vi "FTS Setup Virtual Source.vi"(8 "error in (no error)":errorcluster, 9 "parameters":T1, 10 "type":u16, 11 "specIndex":u16) -> (0 "error out":errorcluster, 1 "parameters out":T1, 3 "function return":i32)   [LabVIEW 2010, in "FTSLib.lvlib"]
doc: "int __cdecl FTS_SetupVirtualSource(unsigned short specIndex, VIRTUAL_SOURCE_TYPE type, virtual_source_parameter_t *parameters);"
uses:
  FTSLib.lvlib
  FTSLib.dll
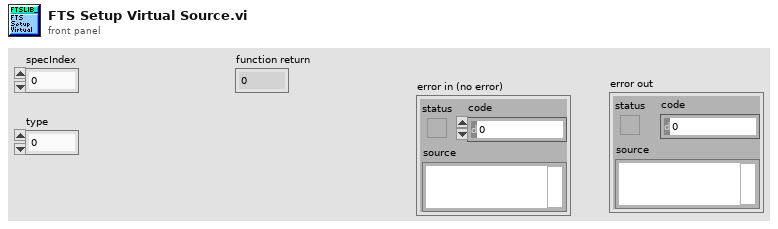
[diagram p1: front panel]
types:
  T1 = cluster{"peakNum":u32, "@dummy control@":i8, "@dummy control@":i8, "@dummy control@":i8, "@dummy control@":i8, "centerWavelength_nm[0]":dbl, "centerWavelength_nm[1]":dbl, "centerWavelength_nm[2]":dbl, "centerWavelength_nm[3]":dbl, "centerWavelength_nm[4]":dbl, "centerWavelength_nm[5]":dbl, "centerWavelength_nm[6]":dbl, "centerWavelength_nm[7]":dbl, "centerWavelength_nm[8]":dbl, "centerWavelength_nm[9]":dbl, "centerWavelength_nm[10]":dbl, "centerWavelength_nm[11]":dbl, "centerWavelength_nm[12]":dbl, "centerWavelength_nm[13]":dbl, "centerWavelength_nm[14]":dbl, "centerWavelength_nm[15]":dbl, "centerWavelength_nm[16]":dbl, "centerWavelength_nm[17]":dbl, "centerWavelength_nm[18]":dbl, "centerWavelength_nm[19]":dbl, "centerWavelength_nm[20]":dbl, "centerWavelength_nm[21]":dbl, "centerWavelength_nm[22]":dbl, "centerWavelength_nm[23]":dbl, "centerWavelength_nm[24]":dbl, "centerWavelength_nm[25]":dbl, "centerWavelength_nm[26]":dbl, "centerWavelength_nm[27]":dbl, "centerWavelength_nm[28]":dbl, "centerWavelength_nm[29]":dbl, "centerWavelength_nm[30]":dbl, "centerWavelength_nm[31]":dbl, "centerWavelength_nm[32]":dbl, "centerWavelength_nm[33]":dbl, "centerWavelength_nm[34]":dbl, "centerWavelength_nm[35]":dbl, "centerWavelength_nm[36]":dbl, "centerWavelength_nm[37]":dbl, "centerWavelength_nm[38]":dbl, "centerWavelength_nm[39]":dbl, "centerWavelength_nm[40]":dbl, "centerWavelength_nm[41]":dbl, "centerWavelength_nm[42]":dbl, "centerWavelength_nm[43]":dbl, "centerWavelength_nm[44]":dbl, "centerWavelength_nm[45]":dbl, "centerWavelength_nm[46]":dbl, "centerWavelength_nm[47]":dbl, "centerWavelength_nm[48]":dbl, "centerWavelength_nm[49]":dbl, "centerWavelength_nm[50]":dbl, "centerWavelength_nm[51]":dbl, "centerWavelength_nm[52]":dbl, "centerWavelength_nm[53]":dbl, "centerWavelength_nm[54]":dbl, "centerWavelength_nm[55]":dbl, "centerWavelength_nm[56]":dbl, "centerWavelength_nm[57]":dbl, "centerWavelength_nm[58]":dbl, "centerWavelength_nm[59]":dbl, "centerWavelength_nm[60]":dbl, "centerWavelength_nm[61]":dbl, "centerWavelength_nm[62]":dbl, "centerWavelength_nm[63]":dbl, "fwhm_nm[0]":dbl, "fwhm_nm[1]":dbl, "fwhm_nm[2]":dbl, "fwhm_nm[3]":dbl, "fwhm_nm[4]":dbl, "fwhm_nm[5]":dbl, "fwhm_nm[6]":dbl, "fwhm_nm[7]":dbl, "fwhm_nm[8]":dbl, "fwhm_nm[9]":dbl, "fwhm_nm[10]":dbl, "fwhm_nm[11]":dbl, "fwhm_nm[12]":dbl, "fwhm_nm[13]":dbl, "fwhm_nm[14]":dbl, "fwhm_nm[15]":dbl, "fwhm_nm[16]":dbl, "fwhm_nm[17]":dbl, "fwhm_nm[18]":dbl, "fwhm_nm[19]":dbl, "fwhm_nm[20]":dbl, "fwhm_nm[21]":dbl, "fwhm_nm[22]":dbl, "fwhm_nm[23]":dbl, "fwhm_nm[24]":dbl, "fwhm_nm[25]":dbl, "fwhm_nm[26]":dbl, "fwhm_nm[27]":dbl, "fwhm_nm[28]":dbl, "fwhm_nm[29]":dbl, "fwhm_nm[30]":dbl, "fwhm_nm[31]":dbl, "fwhm_nm[32]":dbl, "fwhm_nm[33]":dbl, "fwhm_nm[34]":dbl, "fwhm_nm[35]":dbl, "fwhm_nm[36]":dbl, "fwhm_nm[37]":dbl, "fwhm_nm[38]":dbl, "fwhm_nm[39]":dbl, "fwhm_nm[40]":dbl, "fwhm_nm[41]":dbl, "fwhm_nm[42]":dbl, "fwhm_nm[43]":dbl, "fwhm_nm[44]":dbl, "fwhm_nm[45]":dbl, "fwhm_nm[46]":dbl, "fwhm_nm[47]":dbl, "fwhm_nm[48]":dbl, "fwhm_nm[49]":dbl, "fwhm_nm[50]":dbl, "fwhm_nm[51]":dbl, "fwhm_nm[52]":dbl, "fwhm_nm[53]":dbl, "fwhm_nm[54]":dbl, "fwhm_nm[55]":dbl, "fwhm_nm[56]":dbl, "fwhm_nm[57]":dbl, "fwhm_nm[58]":dbl, "fwhm_nm[59]":dbl, "fwhm_nm[60]":dbl, "fwhm_nm[61]":dbl, "fwhm_nm[62]":dbl, "fwhm_nm[63]":dbl, "peakAmplitude[0]":dbl, "peakAmplitude[1]":dbl, "peakAmplitude[2]":dbl, "peakAmplitude[3]":dbl, "peakAmplitude[4]":dbl, "peakAmplitude[5]":dbl, "peakAmplitude[6]":dbl, "peakAmplitude[7]":dbl, "peakAmplitude[8]":dbl, "peakAmplitude[9]":dbl, "peakAmplitude[10]":dbl, "peakAmplitude[11]":dbl, "peakAmplitude[12]":dbl, "peakAmplitude[13]":dbl, "peakAmplitude[14]":dbl, "peakAmplitude[15]":dbl, "peakAmplitude[16]":dbl, "peakAmplitude[17]":dbl, "peakAmplitude[18]":dbl, "peakAmplitude[19]":dbl, "peakAmplitude[20]":dbl, "peakAmplitude[21]":dbl, "peakAmplitude[22]":dbl, "peakAmplitude[23]":dbl, "peakAmplitude[24]":dbl, "peakAmplitude[25]":dbl, "peakAmplitude[26]":dbl, "peakAmplitude[27]":dbl, "peakAmplitude[28]":dbl, "peakAmplitude[29]":dbl, "peakAmplitude[30]":dbl, "peakAmplitude[31]":dbl, "peakAmplitude[32]":dbl, "peakAmplitude[33]":dbl, "peakAmplitude[34]":dbl, "peakAmplitude[35]":dbl, "peakAmplitude[36]":dbl, "peakAmplitude[37]":dbl, "peakAmplitude[38]":dbl, "peakAmplitude[39]":dbl, "peakAmplitude[40]":dbl, "peakAmplitude[41]":dbl, "peakAmplitude[42]":dbl, "peakAmplitude[43]":dbl, "peakAmplitude[44]":dbl, "peakAmplitude[45]":dbl, "peakAmplitude[46]":dbl, "peakAmplitude[47]":dbl, "peakAmplitude[48]":dbl, "peakAmplitude[49]":dbl, "peakAmplitude[50]":dbl, "peakAmplitude[51]":dbl, "peakAmplitude[52]":dbl, "peakAmplitude[53]":dbl, "peakAmplitude[54]":dbl, "peakAmplitude[55]":dbl, "peakAmplitude[56]":dbl, "peakAmplitude[57]":dbl, "peakAmplitude[58]":dbl, "peakAmplitude[59]":dbl, "peakAmplitude[60]":dbl, "peakAmplitude[61]":dbl, "peakAmplitude[62]":dbl, "peakAmplitude[63]":dbl}
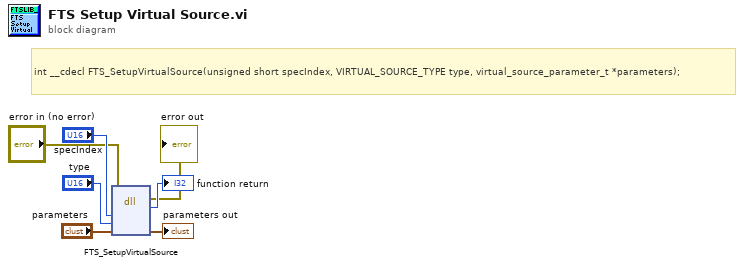
[diagram p0: block diagram]
diagram:
  # "int __cdecl FTS_SetupVirtualSource(unsigned short specIndex, VIRTUAL_SOURCE_TYPE type, virtual_source_parameter_t *parameters);"
  n1 = dll-call lib="FTSLib.*" fn="FTS_SetupVirtualSource"(error in="error in (no error)", "specIndex"="specIndex", "type"="type", "parameters"="parameters") -> (error out=→"error out":errorcluster, →"function return":i32, "parameters"=→"parameters out":T1)  [unwired: 4 in, 1 out]
